vi "Temp LED test.vi"(0 "GEA2 Reference In":refnum<k24>, 5 "Standalone?":bool, 11 "Error In":errorcluster) -> (4 "GEA2 Reference Out":refnum<k24>, 6 "Temp":string="TAP COLD", 10 "Pass/Fail?":bool, 15 "Error Out":errorcluster)   [LabVIEW 2016]
uses:
  Q:/Common/DLLs/GEA3/GeaCommunication.dll
  Common/DLLs/GEA3/GeaCommunication.dll
  Common/LabVIEW GEA2 Toolkit/LabVIEW_GEA2_Toolkit.lvlibp/type defs/ERD Read Data In.ctl
  Common/LabVIEW GEA2 Toolkit/LabVIEW_GEA2_Toolkit.lvlibp/type defs/Data Type.ctl
  Common/LabVIEW GEA2 Toolkit/LabVIEW_GEA2_Toolkit.lvlibp/type defs/Source_Destination.ctl
  Display/controls/HEUI_Display.ctl
  Display/controls/Cycle Selection Enum.ctl
  Display/controls/Stain Enum.ctl
  Display/controls/Temp Enum.ctl
  Display/controls/Soil Enum.ctl
  Display/controls/Spin Enum.ctl
  Display/controls/750 Status Enum.ctl
  Display/controls/HEUI_Display_Care.ctl
  Common/LabVIEW GEA2 Toolkit/LabVIEW_GEA2_Toolkit.lvlibp
  Projects/TL27.lvlib
panel:
  out "Raw Data Out":string
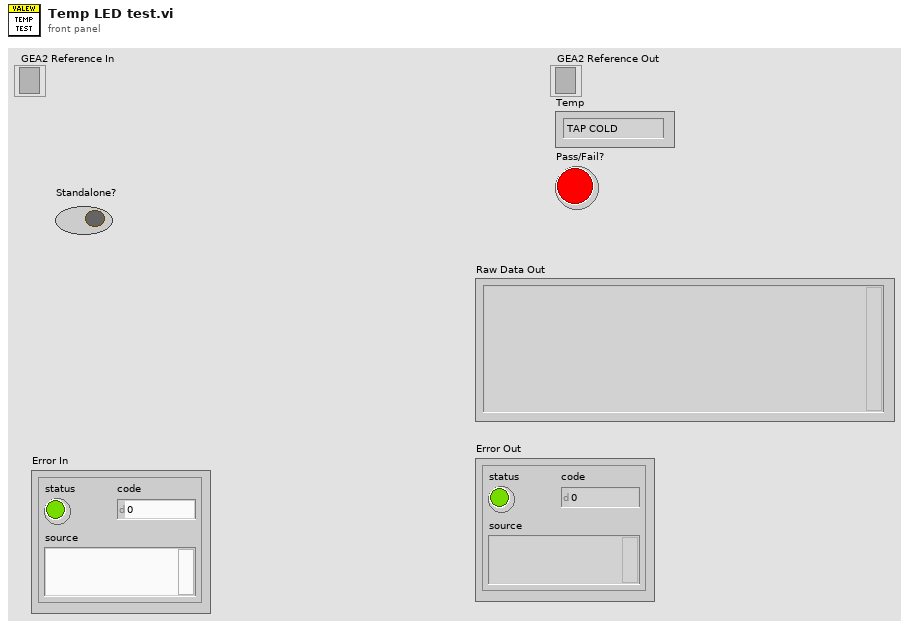
[diagram p1: front panel]
types:
  T1 = typedef "LabVIEW_GEA2_Toolkit.lvlibp/Source_Destination.ctl" = cluster{"Source":u8, "Destination":u8}
  T2 = typedef "LabVIEW_GEA2_Toolkit.lvlibp/ERD Read Data In.ctl" = cluster{"ERD Number":u16, "Data Type":T3}
  T3 = typedef "LabVIEW_GEA2_Toolkit.lvlibp/Data Type.ctl" = enum16{"string", "boolean", "uint8_t", "uint16_t", "uint32_t", "uint64_t", "int8_t", "int16_t", "int32_t", "int64_t"}
  T4 = typedef "TL27.lvlib/HEUI_Display_Care.ctl" = cluster{"SSD":bool, "Cycle Selection":bool, "Stain Selection":bool, "Temp Level":bool, "Soil Level":bool, "Spin Level":bool, "750 Status":bool, "Start":bool, "Pause/WiFi":bool, "Lock Controls":bool, "Lid Lock":bool, "Extra Rinse":bool, "Deep Rinse":bool, "Auto Soak":bool, "Warm Rinse":bool, "Deep Fill":bool, "My Cycle":bool, "Delay Wash":bool, "Spin Stop":bool, "Delay":bool, "Fill":bool, "Soak":bool, "Wash":bool, "Rinse":bool, "Spin":bool}
  T5 = typedef "TL27.lvlib/HEUI_Display.ctl" = cluster{"SSD":string, "Cycle Selection":T6, "Stain Selection":T7, "Temp Level":T8, "Soil Level":T9, "Spin Level":T10, "750 Status":T11, "Start":bool, "Pause/WiFi":bool, "Lock Controls":bool, "Lid Lock":bool, "Extra Rinse":bool, "Deep Rinse":bool, "Auto Soak":bool, "Warm Rinse":bool, "Deep Fill":bool, "My Cycle":bool, "Delay Wash":bool, "Spin Stop":bool, "Delay":bool, "Fill":bool, "Soak":bool, "Wash":bool, "Rinse":bool, "Spin":bool}
  T6 = typedef "TL27.lvlib/Cycle Selection Enum.ctl" = enum16{"Colors", "Easy Care", "Delicates", "Hand Wash", "Active Wear", "Speed Wash", "Rinse and Spin", "Drain and Spin", "Basket Clean", "Jeans", "Heavy Duty", "Bulky Items", "Towels", "Whites", "Off", "*Incorrect*"}
  T7 = typedef "TL27.lvlib/Stain Enum.ctl" = enum16{"Tomato", "Wine", "Blood", "Grass", "Dirt", "Off", "*Incorrect*"}
  T8 = typedef "TL27.lvlib/Temp Enum.ctl" = enum16{"Hot", "Warm", "Colors", "Cool", "Cold", "Tap Cold", "Off", "*Incorrect*"}
  T9 = typedef "TL27.lvlib/Soil Enum.ctl" = enum16{"Extra Heavy", "Heavy", "Normal", "Light", "Off", "*Incorrect*"}
  T10 = typedef "TL27.lvlib/Spin Enum.ctl" = enum16{"Max Spin", "More Spin", "Normal Spin", "No Spin", "Off", "*Incorrect*"}
  T11 = typedef "TL27.lvlib/750 Status Enum.ctl" = enum16{"Fill", "Wash", "Rinse", "Spin", "Off", "*Incorrect*"}
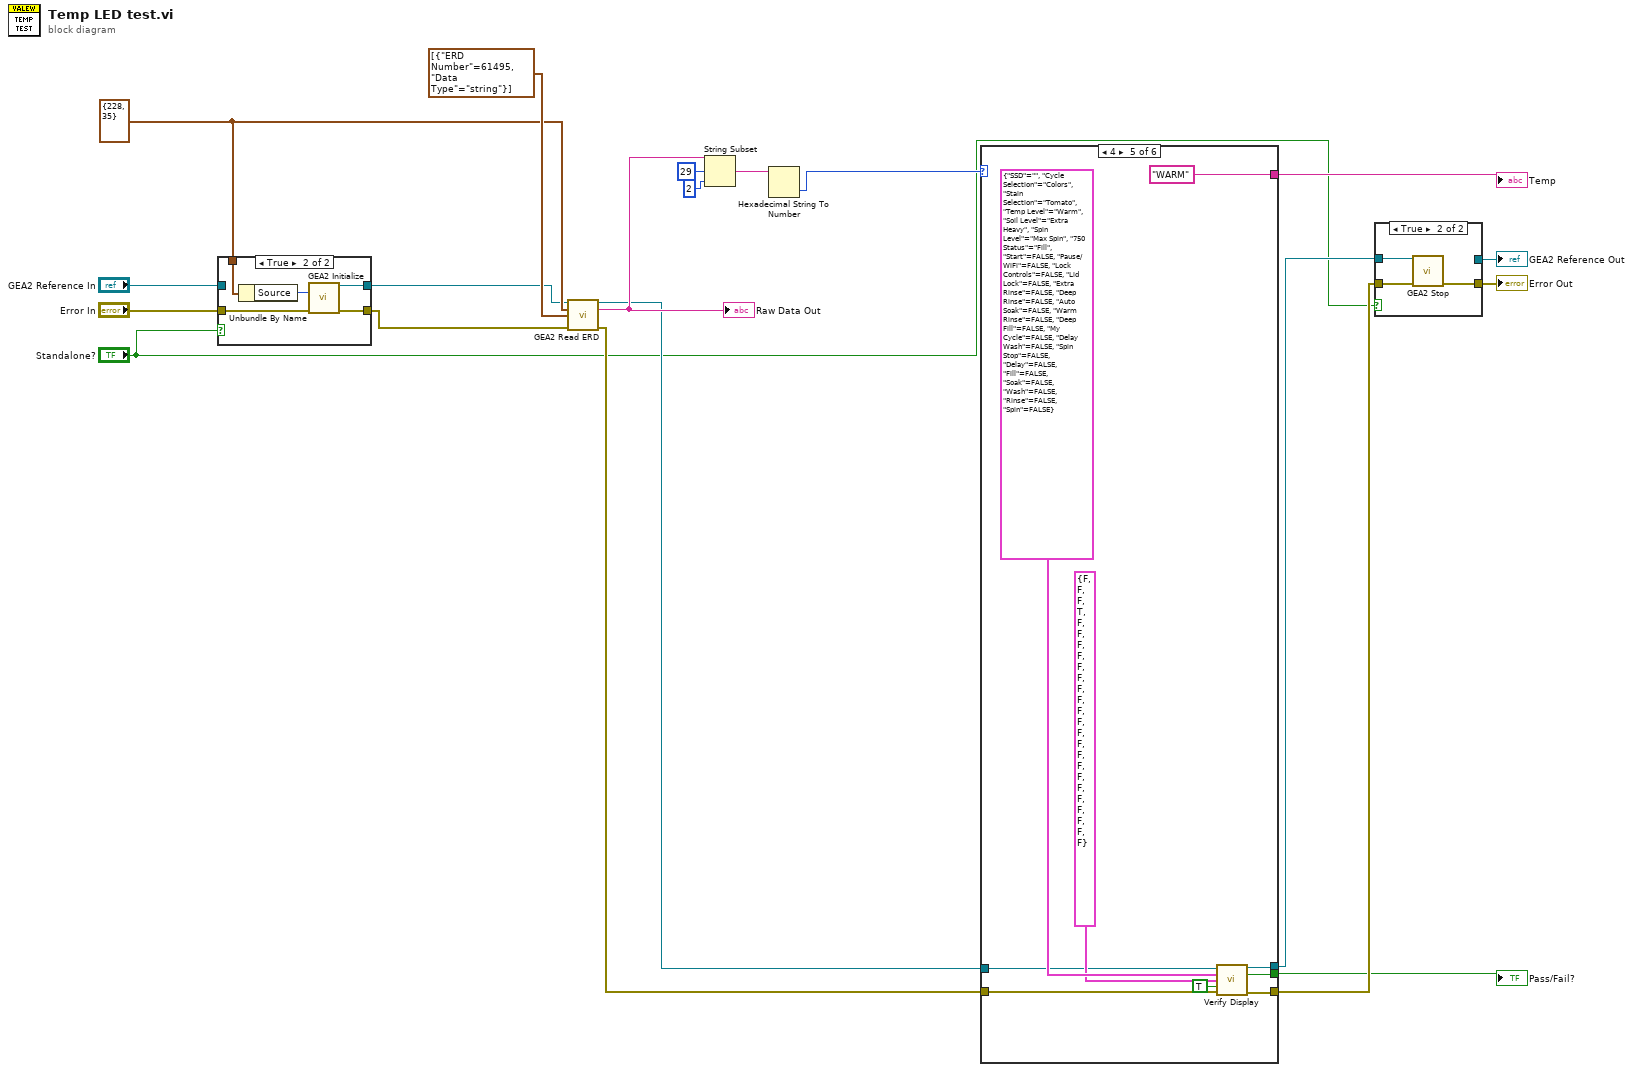
[diagram p0: block diagram]
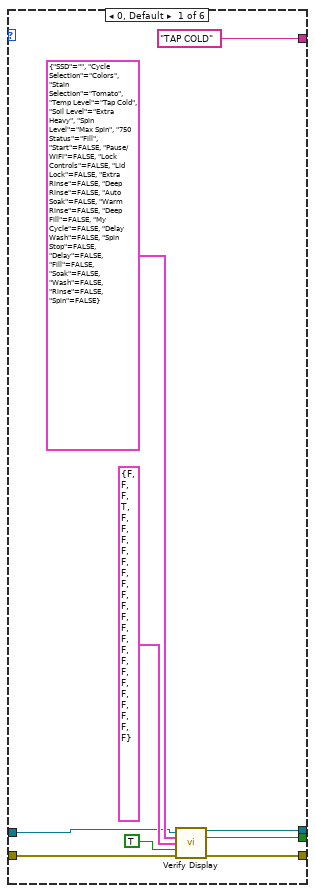
[diagram p2: hidden frame]
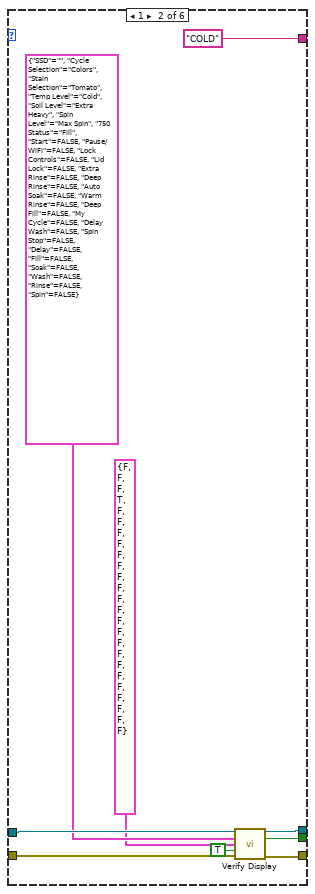
[diagram p3: hidden frame]
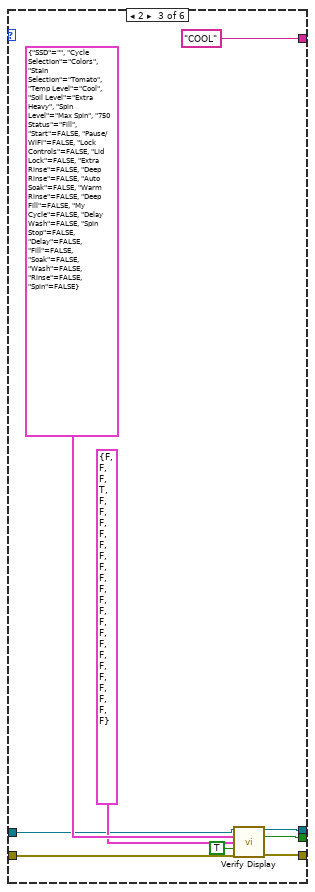
[diagram p4: hidden frame]
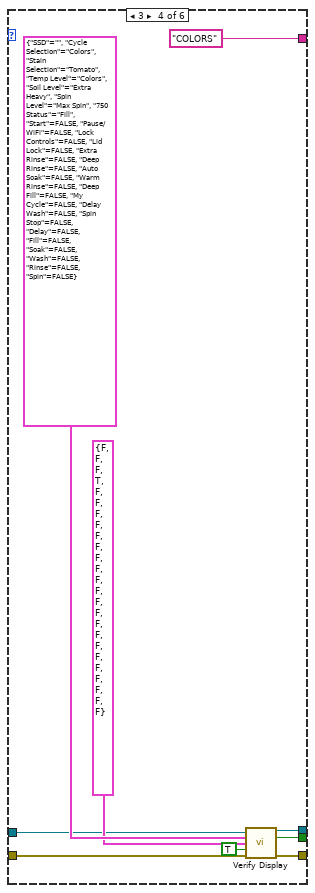
[diagram p5: hidden frame]
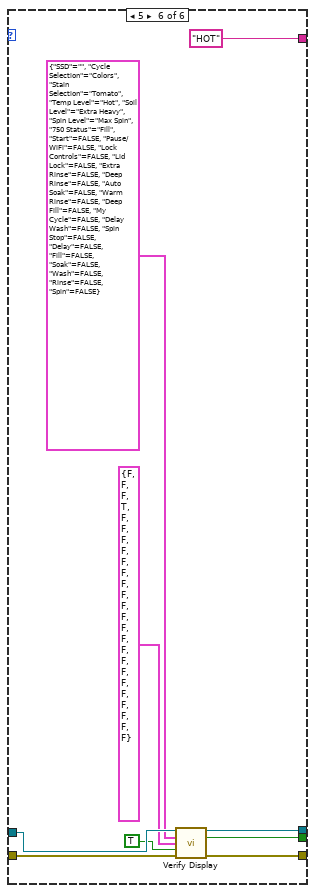
[diagram p6: hidden frame]
diagram:
  w17 = T1 {"Source"=228, "Destination"=35} ("GEA Inputs")
  n1 = case shown="True" "Standalone?" {
    tunnel: "Error In" -> [w21 w27]
    tunnel: [w21 w26] -> w15
    tunnel: "GEA2 Reference In" -> [w22 _]
    tunnel: [w22 w25] -> w16
    tunnel: w17 -> [_ w23]
    frame False {
    }
    frame True {
      n2 = Unbundle By Name(w23) -> ("Source"=w24:u8)
      n3 = call "GEA2 Initialize.vi"("Source Address"=w24, "error in"=w27) -> ("GEA2 Reference Out"=w25:refnum<k24>, "error out"=w26:errorcluster)  [unwired: 11 in, 1 out]
    }
  }
  n4 = call "GEA2 Read ERD.vi"("GEA2 Reference In"=w16, "GEA Inputs"=w17, "Read ERD List"=T2[] [{"ERD Number"=61495, "Data Type"=enum."string"}], "Error In"=w15) -> ("GEA2 Reference Out"=w6:refnum<k24>, "Raw Data Out"=w10:string, "Error Out"=w4:errorcluster)  [unwired: 8 in, 1 out]
  "Raw Data Out" <- w10
  n5 = String Subset(string=w10, offset (0)=29, length (rest)=2 ("length (rest)")) -> (substring=w9:string)
  n6 = Hexadecimal String To Number(string=w9) -> (number=w8:u32)  [unwired: 2 in, 1 out]
  n7 = case shown="4" w8 {
    tunnel: ["TAP COLD" "COLD" "COOL" "COLORS" "WARM" "HOT"] -> w7
    tunnel: w6 -> [w33 w41 w48 w57 w66 w80]
    tunnel: [w30 w44 w53 w62 w71 w79] -> w5
    tunnel: w4 -> [w32 w40 w47 w56 w65 w78]
    tunnel: [w29 w42 w51 w60 w69 w77] -> w3
    tunnel: [w28 w43 w52 w61 w70 w73] -> w2
    frame 0, Default {
      n8 = call "Verify Display.vi"("GEA2 Reference In"=w33, "Expected LEDs"=T5 {"SSD"="", "Cycle Selection"=enum."Colors", "Stain Selection"=enum."Tomato", "Temp Level"=enum."Tap Cold", "Soil Level"=enum."Extra Heavy", "Spin Level"=enum."Max Spin", "750 Status"=enum."Fill", "Start"=FALSE, "Pause/WiFi"=FALSE, "Lock Controls"=FALSE, "Lid Lock"=FALSE, "Extra Rinse"=FALSE, "Deep Rinse"=FALSE, "Auto Soak"=FALSE, "Warm Rinse"=FALSE, "Deep Fill"=FALSE, "My Cycle"=FALSE, "Delay Wash"=FALSE, "Spin Stop"=FALSE, "Delay"=FALSE, "Fill"=FALSE, "Soak"=FALSE, "Wash"=FALSE, "Rinse"=FALSE, "Spin"=FALSE}, "Care?"=T4 {"SSD"=FALSE, "Cycle Selection"=FALSE, "Stain Selection"=FALSE, "Temp Level"=TRUE, "Soil Level"=FALSE, "Spin Level"=FALSE, "750 Status"=FALSE, "Start"=FALSE, "Pause/WiFi"=FALSE, "Lock Controls"=FALSE, "Lid Lock"=FALSE, "Extra Rinse"=FALSE, "Deep Rinse"=FALSE, "Auto Soak"=FALSE, "Warm Rinse"=FALSE, "Deep Fill"=FALSE, "My Cycle"=FALSE, "Delay Wash"=FALSE, "Spin Stop"=FALSE, "Delay"=FALSE, "Fill"=FALSE, "Soak"=FALSE, "Wash"=FALSE, "Rinse"=FALSE, "Spin"=FALSE}, "Ignore Brightness?"=TRUE, "Error In"=w32) -> ("GEA2 Reference Out"=w30:refnum<k24>, "Pass/Fail?"=w28:bool, "Error Out"=w29:errorcluster)  [unwired: 7 in, 1 out]
    }
    frame 1 {
      n9 = call "Verify Display.vi"("GEA2 Reference In"=w41, "Expected LEDs"=T5 {"SSD"="", "Cycle Selection"=enum."Colors", "Stain Selection"=enum."Tomato", "Temp Level"=enum."Cold", "Soil Level"=enum."Extra Heavy", "Spin Level"=enum."Max Spin", "750 Status"=enum."Fill", "Start"=FALSE, "Pause/WiFi"=FALSE, "Lock Controls"=FALSE, "Lid Lock"=FALSE, "Extra Rinse"=FALSE, "Deep Rinse"=FALSE, "Auto Soak"=FALSE, "Warm Rinse"=FALSE, "Deep Fill"=FALSE, "My Cycle"=FALSE, "Delay Wash"=FALSE, "Spin Stop"=FALSE, "Delay"=FALSE, "Fill"=FALSE, "Soak"=FALSE, "Wash"=FALSE, "Rinse"=FALSE, "Spin"=FALSE}, "Care?"=T4 {"SSD"=FALSE, "Cycle Selection"=FALSE, "Stain Selection"=FALSE, "Temp Level"=TRUE, "Soil Level"=FALSE, "Spin Level"=FALSE, "750 Status"=FALSE, "Start"=FALSE, "Pause/WiFi"=FALSE, "Lock Controls"=FALSE, "Lid Lock"=FALSE, "Extra Rinse"=FALSE, "Deep Rinse"=FALSE, "Auto Soak"=FALSE, "Warm Rinse"=FALSE, "Deep Fill"=FALSE, "My Cycle"=FALSE, "Delay Wash"=FALSE, "Spin Stop"=FALSE, "Delay"=FALSE, "Fill"=FALSE, "Soak"=FALSE, "Wash"=FALSE, "Rinse"=FALSE, "Spin"=FALSE}, "Ignore Brightness?"=TRUE, "Error In"=w40) -> ("GEA2 Reference Out"=w44:refnum<k24>, "Pass/Fail?"=w43:bool, "Error Out"=w42:errorcluster)  [unwired: 7 in, 1 out]
    }
    frame 2 {
      n10 = call "Verify Display.vi"("GEA2 Reference In"=w48, "Expected LEDs"=T5 {"SSD"="", "Cycle Selection"=enum."Colors", "Stain Selection"=enum."Tomato", "Temp Level"=enum."Cool", "Soil Level"=enum."Extra Heavy", "Spin Level"=enum."Max Spin", "750 Status"=enum."Fill", "Start"=FALSE, "Pause/WiFi"=FALSE, "Lock Controls"=FALSE, "Lid Lock"=FALSE, "Extra Rinse"=FALSE, "Deep Rinse"=FALSE, "Auto Soak"=FALSE, "Warm Rinse"=FALSE, "Deep Fill"=FALSE, "My Cycle"=FALSE, "Delay Wash"=FALSE, "Spin Stop"=FALSE, "Delay"=FALSE, "Fill"=FALSE, "Soak"=FALSE, "Wash"=FALSE, "Rinse"=FALSE, "Spin"=FALSE}, "Care?"=T4 {"SSD"=FALSE, "Cycle Selection"=FALSE, "Stain Selection"=FALSE, "Temp Level"=TRUE, "Soil Level"=FALSE, "Spin Level"=FALSE, "750 Status"=FALSE, "Start"=FALSE, "Pause/WiFi"=FALSE, "Lock Controls"=FALSE, "Lid Lock"=FALSE, "Extra Rinse"=FALSE, "Deep Rinse"=FALSE, "Auto Soak"=FALSE, "Warm Rinse"=FALSE, "Deep Fill"=FALSE, "My Cycle"=FALSE, "Delay Wash"=FALSE, "Spin Stop"=FALSE, "Delay"=FALSE, "Fill"=FALSE, "Soak"=FALSE, "Wash"=FALSE, "Rinse"=FALSE, "Spin"=FALSE}, "Ignore Brightness?"=TRUE, "Error In"=w47) -> ("GEA2 Reference Out"=w53:refnum<k24>, "Pass/Fail?"=w52:bool, "Error Out"=w51:errorcluster)  [unwired: 7 in, 1 out]
    }
    frame 3 {
      n11 = call "Verify Display.vi"("GEA2 Reference In"=w57, "Expected LEDs"=T5 {"SSD"="", "Cycle Selection"=enum."Colors", "Stain Selection"=enum."Tomato", "Temp Level"=enum."Colors", "Soil Level"=enum."Extra Heavy", "Spin Level"=enum."Max Spin", "750 Status"=enum."Fill", "Start"=FALSE, "Pause/WiFi"=FALSE, "Lock Controls"=FALSE, "Lid Lock"=FALSE, "Extra Rinse"=FALSE, "Deep Rinse"=FALSE, "Auto Soak"=FALSE, "Warm Rinse"=FALSE, "Deep Fill"=FALSE, "My Cycle"=FALSE, "Delay Wash"=FALSE, "Spin Stop"=FALSE, "Delay"=FALSE, "Fill"=FALSE, "Soak"=FALSE, "Wash"=FALSE, "Rinse"=FALSE, "Spin"=FALSE}, "Care?"=T4 {"SSD"=FALSE, "Cycle Selection"=FALSE, "Stain Selection"=FALSE, "Temp Level"=TRUE, "Soil Level"=FALSE, "Spin Level"=FALSE, "750 Status"=FALSE, "Start"=FALSE, "Pause/WiFi"=FALSE, "Lock Controls"=FALSE, "Lid Lock"=FALSE, "Extra Rinse"=FALSE, "Deep Rinse"=FALSE, "Auto Soak"=FALSE, "Warm Rinse"=FALSE, "Deep Fill"=FALSE, "My Cycle"=FALSE, "Delay Wash"=FALSE, "Spin Stop"=FALSE, "Delay"=FALSE, "Fill"=FALSE, "Soak"=FALSE, "Wash"=FALSE, "Rinse"=FALSE, "Spin"=FALSE}, "Ignore Brightness?"=TRUE, "Error In"=w56) -> ("GEA2 Reference Out"=w62:refnum<k24>, "Pass/Fail?"=w61:bool, "Error Out"=w60:errorcluster)  [unwired: 7 in, 1 out]
    }
    frame 4 {
      n12 = call "Verify Display.vi"("GEA2 Reference In"=w66, "Expected LEDs"=T5 {"SSD"="", "Cycle Selection"=enum."Colors", "Stain Selection"=enum."Tomato", "Temp Level"=enum."Warm", "Soil Level"=enum."Extra Heavy", "Spin Level"=enum."Max Spin", "750 Status"=enum."Fill", "Start"=FALSE, "Pause/WiFi"=FALSE, "Lock Controls"=FALSE, "Lid Lock"=FALSE, "Extra Rinse"=FALSE, "Deep Rinse"=FALSE, "Auto Soak"=FALSE, "Warm Rinse"=FALSE, "Deep Fill"=FALSE, "My Cycle"=FALSE, "Delay Wash"=FALSE, "Spin Stop"=FALSE, "Delay"=FALSE, "Fill"=FALSE, "Soak"=FALSE, "Wash"=FALSE, "Rinse"=FALSE, "Spin"=FALSE}, "Care?"=T4 {"SSD"=FALSE, "Cycle Selection"=FALSE, "Stain Selection"=FALSE, "Temp Level"=TRUE, "Soil Level"=FALSE, "Spin Level"=FALSE, "750 Status"=FALSE, "Start"=FALSE, "Pause/WiFi"=FALSE, "Lock Controls"=FALSE, "Lid Lock"=FALSE, "Extra Rinse"=FALSE, "Deep Rinse"=FALSE, "Auto Soak"=FALSE, "Warm Rinse"=FALSE, "Deep Fill"=FALSE, "My Cycle"=FALSE, "Delay Wash"=FALSE, "Spin Stop"=FALSE, "Delay"=FALSE, "Fill"=FALSE, "Soak"=FALSE, "Wash"=FALSE, "Rinse"=FALSE, "Spin"=FALSE}, "Ignore Brightness?"=TRUE, "Error In"=w65) -> ("GEA2 Reference Out"=w71:refnum<k24>, "Pass/Fail?"=w70:bool, "Error Out"=w69:errorcluster)  [unwired: 7 in, 1 out]
    }
    frame 5 {
      n13 = call "Verify Display.vi"("GEA2 Reference In"=w80, "Expected LEDs"=T5 {"SSD"="", "Cycle Selection"=enum."Colors", "Stain Selection"=enum."Tomato", "Temp Level"=enum."Hot", "Soil Level"=enum."Extra Heavy", "Spin Level"=enum."Max Spin", "750 Status"=enum."Fill", "Start"=FALSE, "Pause/WiFi"=FALSE, "Lock Controls"=FALSE, "Lid Lock"=FALSE, "Extra Rinse"=FALSE, "Deep Rinse"=FALSE, "Auto Soak"=FALSE, "Warm Rinse"=FALSE, "Deep Fill"=FALSE, "My Cycle"=FALSE, "Delay Wash"=FALSE, "Spin Stop"=FALSE, "Delay"=FALSE, "Fill"=FALSE, "Soak"=FALSE, "Wash"=FALSE, "Rinse"=FALSE, "Spin"=FALSE}, "Care?"=T4 {"SSD"=FALSE, "Cycle Selection"=FALSE, "Stain Selection"=FALSE, "Temp Level"=TRUE, "Soil Level"=FALSE, "Spin Level"=FALSE, "750 Status"=FALSE, "Start"=FALSE, "Pause/WiFi"=FALSE, "Lock Controls"=FALSE, "Lid Lock"=FALSE, "Extra Rinse"=FALSE, "Deep Rinse"=FALSE, "Auto Soak"=FALSE, "Warm Rinse"=FALSE, "Deep Fill"=FALSE, "My Cycle"=FALSE, "Delay Wash"=FALSE, "Spin Stop"=FALSE, "Delay"=FALSE, "Fill"=FALSE, "Soak"=FALSE, "Wash"=FALSE, "Rinse"=FALSE, "Spin"=FALSE}, "Ignore Brightness?"=TRUE, "Error In"=w78) -> ("GEA2 Reference Out"=w79:refnum<k24>, "Pass/Fail?"=w73:bool, "Error Out"=w77:errorcluster)  [unwired: 7 in, 1 out]
    }
  }
  "Temp" <- w7
  "Pass/Fail?" <- w2
  n14 = case shown="True" "Standalone?" {
    tunnel: [w83 w86] -> w13
    tunnel: w3 -> [w83 w85]
    tunnel: w5 -> [w82 w84]
    tunnel: [w82 _] -> w14
    frame False {
    }
    frame True {
      n15 = call "GEA2 Stop.vi"("GEA2 Reference In"=w84, "Error In"=w85) -> ("Error Out"=w86:errorcluster)  [unwired: 13 in]
    }
  }
  "GEA2 Reference Out" <- w14
  "Error Out" <- w13
